vi "QD Dig Grave.vi"(6 "Variant in":variant, 7 "Shift Pressed?":bool, 8 "error in (no error)":errorcluster, 10 "QD Combo Box Ref":refnum<vi>, 11 "QD Launch VI Ref":refnum<vi>) -> (0 "error out":errorcluster, 4 "Variant out":variant)   [LabVIEW 2017, in "Eulogy.lvlib"]
doc: "Digs a grave for the currently selected code. A grave is a Diagram Disable structure with a bookmark for the structure label that includes \"RIP\", the time of death (YYYYMMDD), and the grave digger (programmer). The selected code is placed in the Disabled frame, which will have the \"Corpse\" subdiagram label and a duplicate of the Disabled frame is created for the Enabled frame, which will have the \"Spirit\" subdiagram label. The spirit of the original code, that could be dead, can then be safely refactored.\n\nDefault Shortcut - [G]"
uses:
  Eulogy.lvlib
panel:
  # "Do not change the connector pane of this VI.\n\nSee the block diagram for directions on how to use this template."
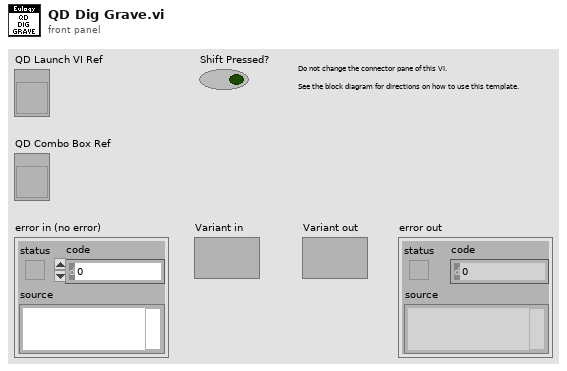
[diagram p1: front panel]
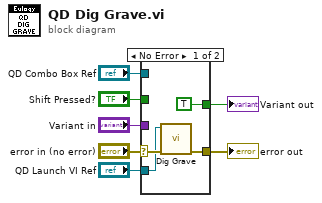
[diagram p0: block diagram]
diagram:
  n1 = case shown="No Error" "error in (no error)" {
    selector: "error in (no error)" -> [w10 w12]
    tunnel: [w11 w12] -> w7
    tunnel: [TRUE _] -> w5
    tunnel: "Variant in" -> [_ _]
    tunnel: "Shift Pressed?" -> [_ _]
    tunnel: "QD Launch VI Ref" -> [w8 _]
    tunnel: "QD Combo Box Ref" -> [_ _]
    frame No Error {
      n2 = call "Dig Grave.vi"("Error In"=w10, "VI In"=w8) -> ("Error Out"=w11:errorcluster)  [unwired: 8 in, 1 out]
    }
    frame Error {
    }
  }
  "error out" <- w7
  "Variant out" <- w5
